vi "Save Error Report V0.50.vi"(3 "Error Message":string, 5 "Error Code (0: No Error)":i32, 6 "Path":path) -> (0 "Written content":string)   [LabVIEW 2021]
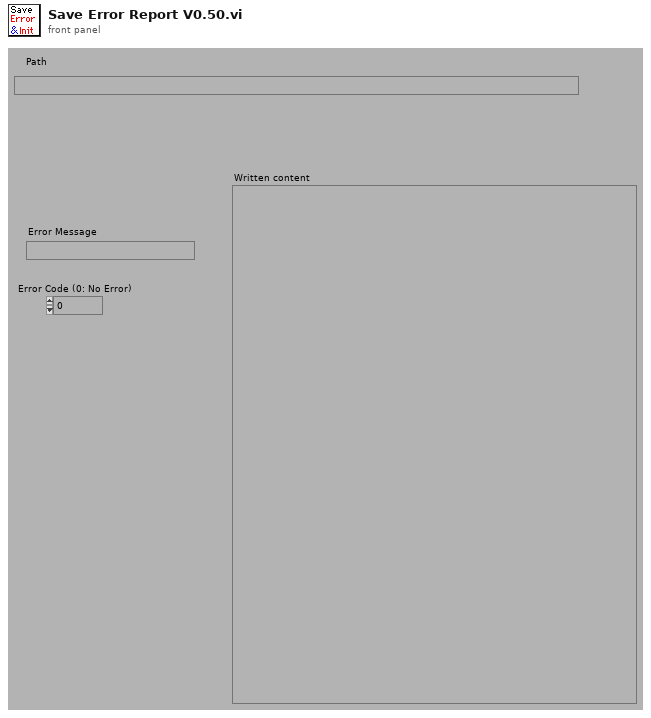
[diagram p1: front panel]
types:
  T1 = enum16{"open", "open or create", "create or replace", "create"}
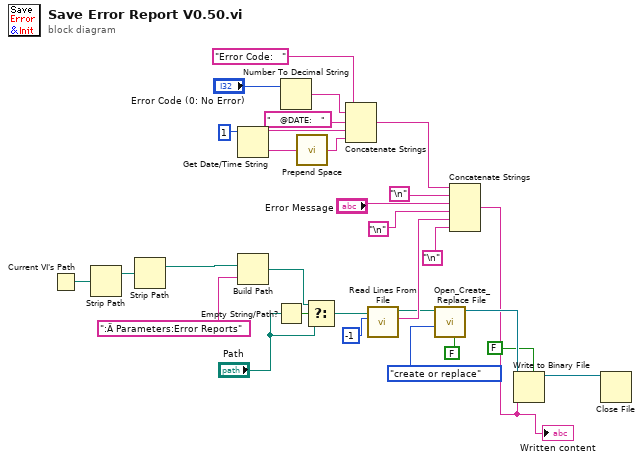
[diagram p0: block diagram]
diagram:
  n1 = Current VI's Path() -> (path=w6:path)
  n2 = Strip Path(path=w6) -> (stripped path=w8:path)  [unwired: 1 out]
  n3 = Strip Path(path=w8) -> (stripped path=w2:path)  [unwired: 1 out]
  n4 = Get Date/Time String(date format (0)=1) -> (date string=w24:string, time string=w26:string)  [unwired: 2 in]
  n5 = Build Path(base path=w2, name or relative path=":Ä Parameters:Error Reports") -> (appended path=w5:path)
  n6 = Empty String/Path?(string/path="Path") -> (empty?=w9:bool)
  n7 = Number To Decimal String(number="Error Code (0: No Error)") -> (decimal integer string=w16:string)  [unwired: 1 in]
  n8 = call "Prepend Space.vi"("Input String"=w26) -> ("Space + Input String"=w25:string)
  n9 = Select(t=w5, s=w9, f="Path") -> (s? t:f=w3:path)
  n10 = Concatenate Strings("Error Code:   ", w16, "   @DATE:   " ("date string"), w24, w25) -> (w13:string)
  n11 = call <vilib>:"Read Lines From File.vi"("file path (dialog if empty)"=w3, "number of lines (all:-1)"=-1) -> ("new file path (Not A Path if cancelled)"=w14:path, "line string"=w20:string)  [unwired: 4 in, 2 out]
  n12 = call <vilib>:"Open_Create_Replace File.vi"("advisory dialog? (display:T)"=FALSE, "function (open:0)"=T1."create or replace", "file path"=w14) -> ("refnum"=w22:refnum<file>)  [unwired: 5 in, 3 out]
  n13 = Concatenate Strings(w13, "\n", "Error Message", "\n", w20, "\n") -> (w19:string)
  "Written content" <- w19
  n14 = Write to Binary File(file (use dialog)=w22, data=w19, 5:FALSE ("prepend array or string size? (T)")) -> (refnum out=w29:refnum<file>)  [unwired: 3 in, 2 out]
  n15 = Close File(refnum=w29) -> ()  [unwired: 1 in, 2 out]
